vi "Autonomous Independent.vi"() -> ()   [LabVIEW 2013]
doc: "This VI is called when autonomous begins, and will automatically be terminated when autonomous ends. You can carry out timed or sensor driven robot movement independently without needing to return to the caller."
uses:
  Begin/Global Refnums.vi
  Begin/Global Variables.vi
  <vilib>/Rock Robotics/WPI/DriverStation/DriverStationLCD/WPI_DriverStationLCDLCDLine.ctl
panel:
  out "Index 2":i32
  # "Be sure to right-click and choose Data Operations>>Make Current Value default if you want to save the array values with the VI"
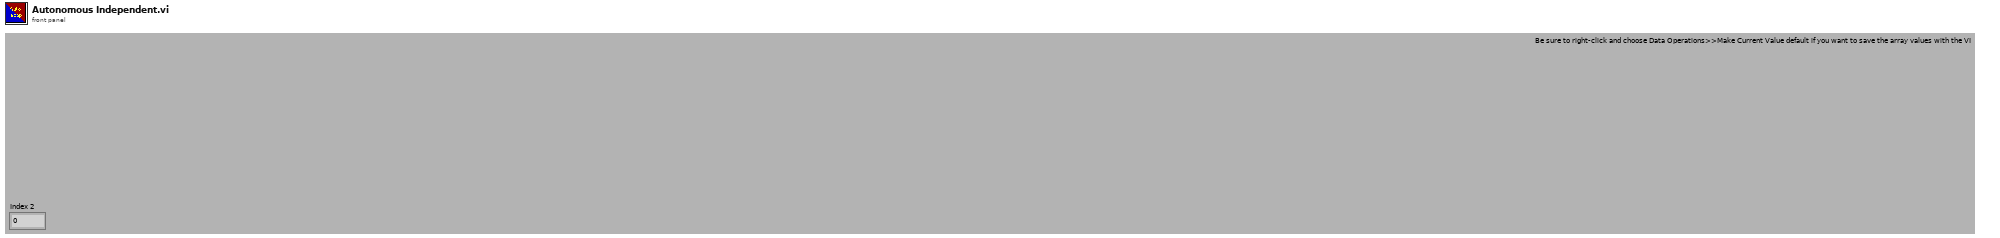
[diagram p1: front panel]
types:
  T1 = typedef "WPI_DriverStationLCDLCDLine.ctl" = enum16{"Main - Line 1", "User - Line 2", "User - Line 3", "User - Line 4", "User - Line 5", "User - Line 6"}
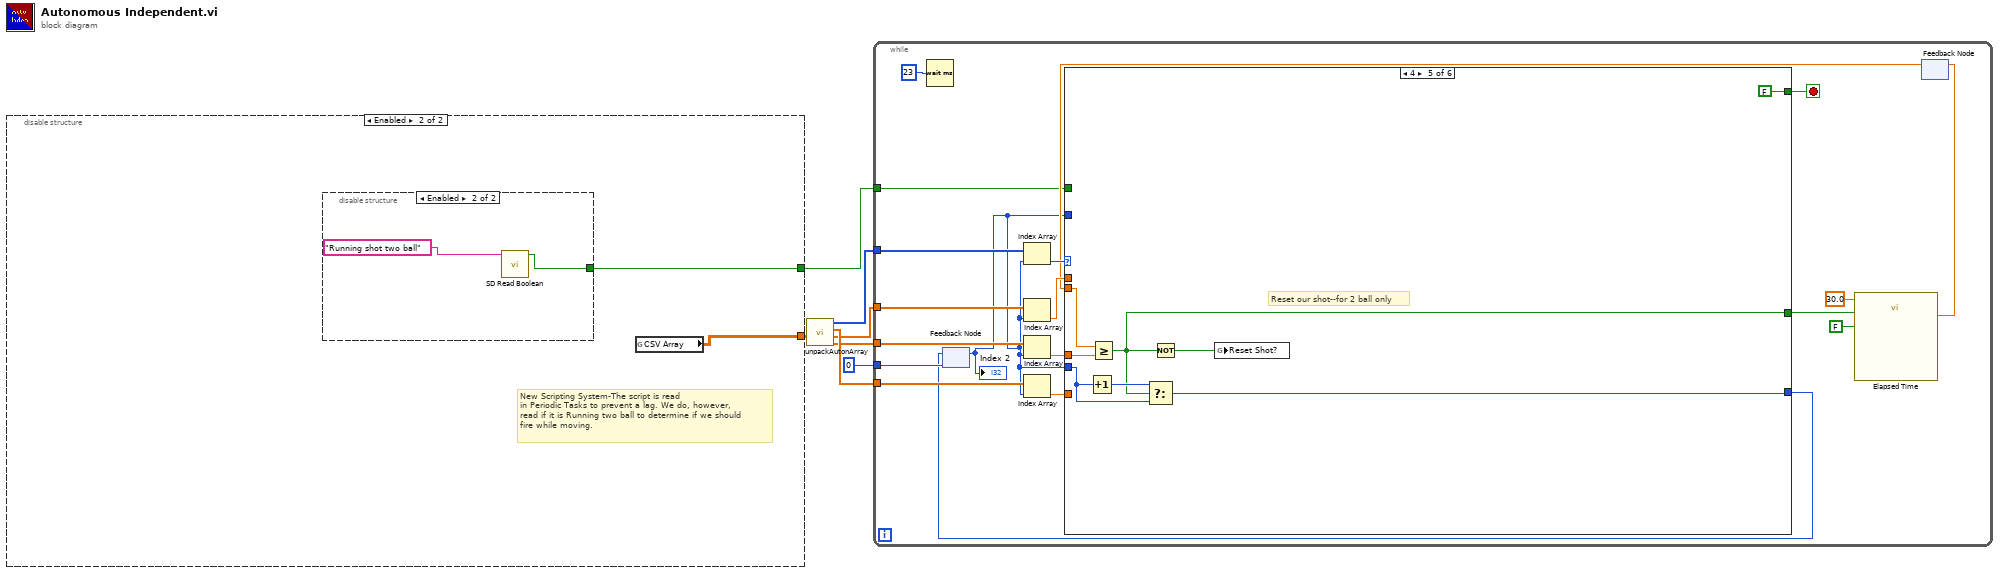
[diagram p0: block diagram]
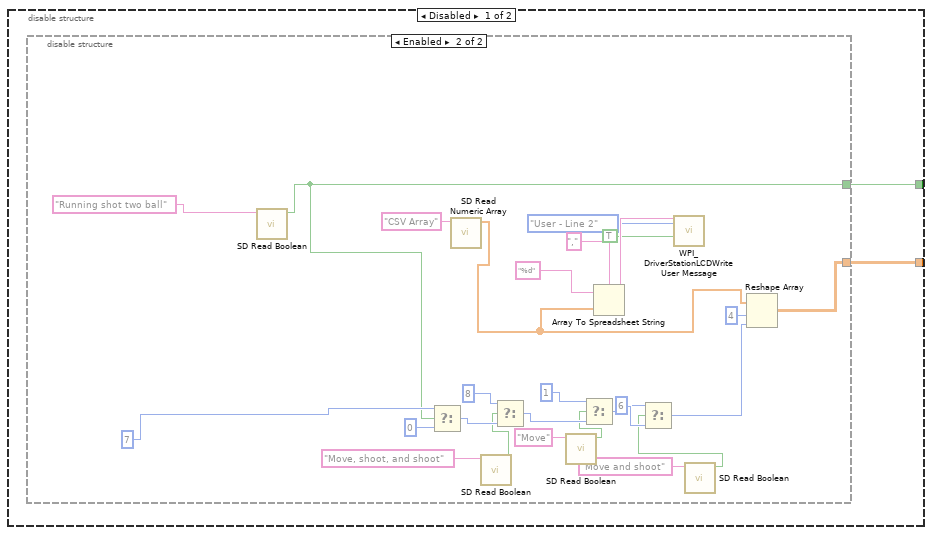
[diagram p2: hidden frame]
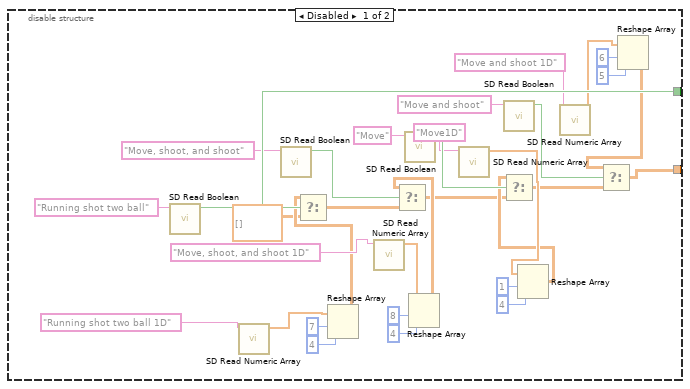
[diagram p3: hidden frame]
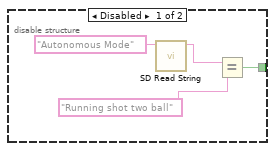
[diagram p4: hidden frame]
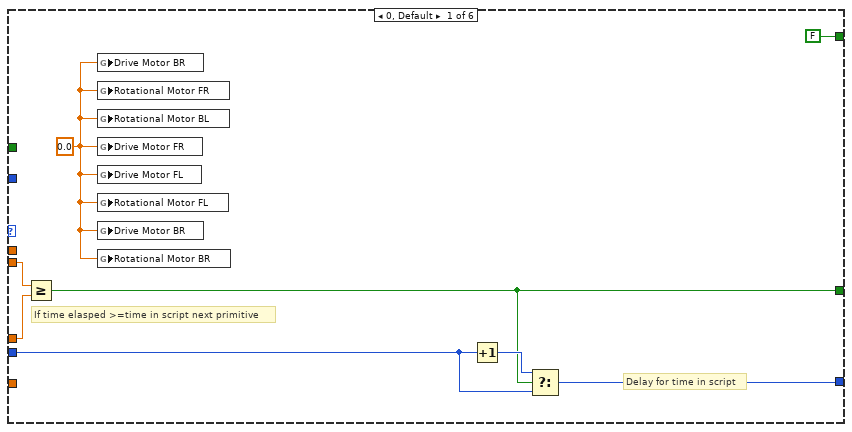
[diagram p5: hidden frame]
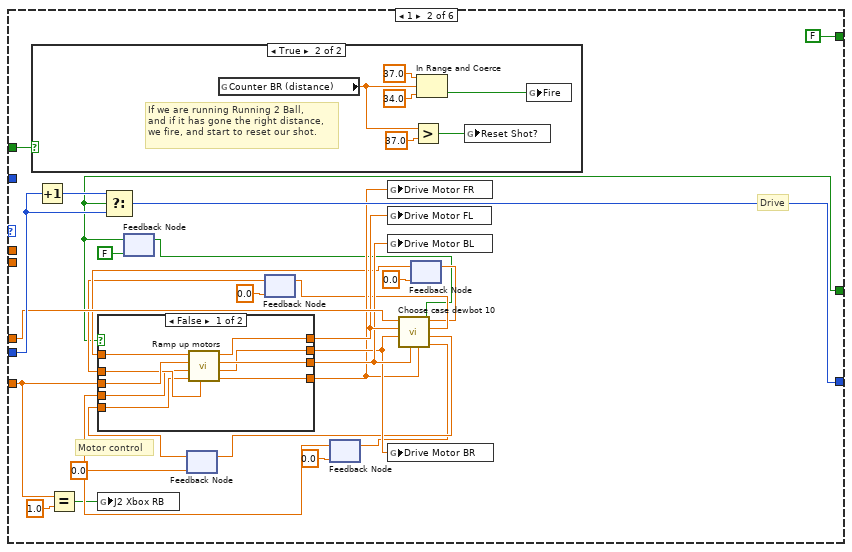
[diagram p6: hidden frame]
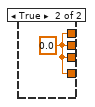
[diagram p8: hidden frame]
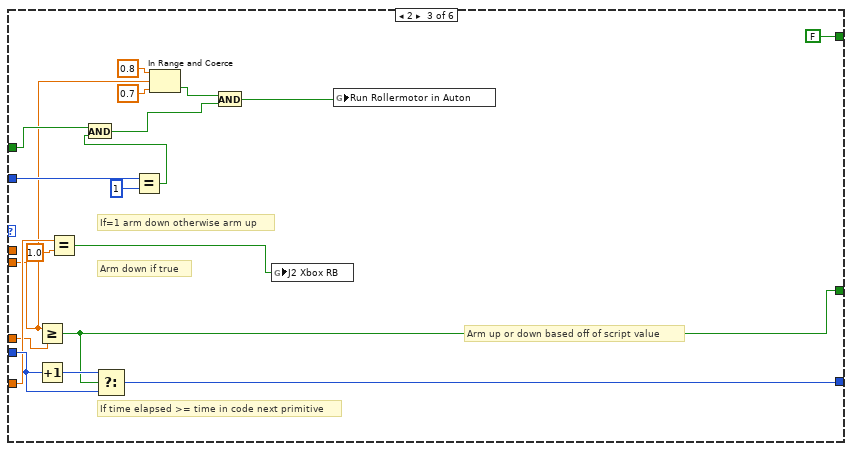
[diagram p9: hidden frame]
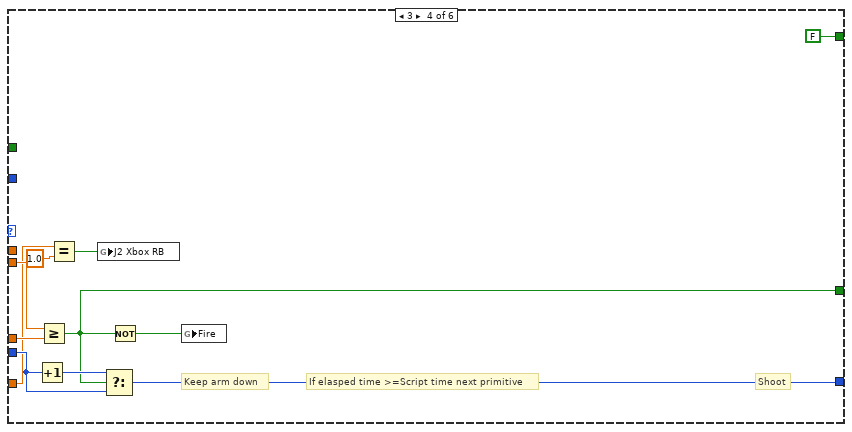
[diagram p10: hidden frame]
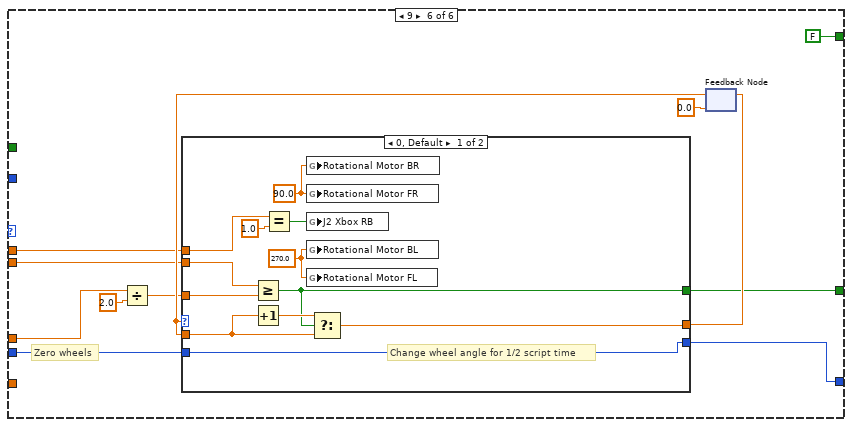
[diagram p11: hidden frame]
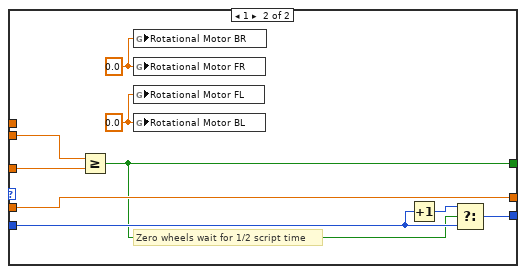
[diagram p12: hidden frame]
diagram:
  n1 = disable-structure shown="Enabled" {
    disable-tunnel: [w9 w69] -> w2
    disable-tunnel: [w8 w70] -> w1
    frame Disabled {
      n2 = disable-structure shown="Enabled" {
        disable-tunnel: [w42 w57] -> w9
        disable-tunnel: [w11 w49] -> w8
        frame Disabled {
          n3 = call <vilib>:"SD Read Boolean.vi"("Name"="Running shot two ball") -> ("Boolean"=w42:bool)  [unwired: 8 in, 2 out]
          n4 = call <vilib>:"SD Read Numeric Array.vi"("Name"="Running shot two ball 1D") -> ("Numeric Array"=w15:dbl[])  [unwired: 8 in, 2 out]
          n5 = call <vilib>:"SD Read Boolean.vi"("Name"="Move, shoot, and shoot") -> ("Boolean"=w35:bool)  [unwired: 8 in, 2 out]
          n6 = Reshape Array(w15, 7 ("dimension size"), 4 ("dimension size")) -> (w14:dbl[][])
          n7 = Select(t=w14, s=w42, f=dbl[][] []) -> (s? t:f=w13:dbl[][])
          n8 = call <vilib>:"SD Read Numeric Array.vi"("Name"="Move, shoot, and shoot 1D") -> ("Numeric Array"=w18:dbl[])  [unwired: 8 in, 2 out]
          n9 = call <vilib>:"SD Read Boolean.vi"("Name"="Move") -> ("Boolean"=w39:bool)  [unwired: 8 in, 2 out]
          n10 = Reshape Array(w18, 8 ("dimension size"), 4 ("dimension size")) -> (w17:dbl[][])
          n11 = Select(t=w17, s=w35, f=w13) -> (s? t:f=w16:dbl[][])
          n12 = call <vilib>:"SD Read Numeric Array.vi"("Name"="Move1D") -> ("Numeric Array"=w20:dbl[])  [unwired: 8 in, 2 out]
          n13 = call <vilib>:"SD Read Boolean.vi"("Name"="Move and shoot") -> ("Boolean"=w38:bool)  [unwired: 8 in, 2 out]
          n14 = Reshape Array(w20, 1 ("dimension size"), 4 ("dimension size")) -> (w19:dbl[][])
          n15 = Select(t=w19, s=w39, f=w16) -> (s? t:f=w12:dbl[][])
          n16 = call <vilib>:"SD Read Numeric Array.vi"("Name"="Move and shoot 1D") -> ("Numeric Array"=w30:dbl[])  [unwired: 8 in, 2 out]
          n17 = Reshape Array(w30, 6 ("dimension size"), 5 ("dimension size")) -> (w27:dbl[][])
          n18 = Select(t=w27, s=w38, f=w12) -> (s? t:f=w11:dbl[][])
        }
        frame Enabled {
          n19 = call <vilib>:"SD Read Boolean.vi"("Name"="Running shot two ball") -> ("Boolean"=w57:bool)  [unwired: 8 in, 2 out]
          n20 = Select(t=7 ("dimension size"), s=w57, f=0) -> (s? t:f=w63:i32)
          n21 = call <vilib>:"SD Read Numeric Array.vi"("Name"="CSV Array") -> ("Numeric Array"=w44:dbl[])  [unwired: 8 in, 2 out]
          n22 = call <vilib>:"SD Read Boolean.vi"("Name"="Move, shoot, and shoot") -> ("Boolean"=w52:bool)  [unwired: 8 in, 2 out]
          n23 = Select(t=8 ("dimension size"), s=w52, f=w63) -> (s? t:f=w61:i32)
          n24 = call <vilib>:"SD Read Boolean.vi"("Name"="Move") -> ("Boolean"=w54:bool)  [unwired: 8 in, 2 out]
          n25 = Select(t=1 ("dimension size"), s=w54, f=w61) -> (s? t:f=w60:i32)
          n26 = Array To Spreadsheet String(delimiter (Tab)=",", array=w44, 3:"%d" ("format string")) -> (spreadsheet string=w48:string)
          n27 = call <vilib>:"WPI_DriverStationLCDWrite User Message.vi"("line text"=w48, "line"=WPI_DriverStationLCDLCDLine."User - Line 2", "clear line before write (T)"=TRUE) -> ()  [unwired: 12 in, 1 out]
          n28 = call <vilib>:"SD Read Boolean.vi"("Name"="Move and shoot") -> ("Boolean"=w50:bool)  [unwired: 8 in, 2 out]
          n29 = Select(t=6, s=w50, f=w60) -> (s? t:f=w56:i32)
          n30 = Reshape Array(w44, 4 ("dimension size"), w56) -> (w49:dbl[][])
        }
      }
    }
    frame Enabled {
      # "New Scripting System-The script is read \nin Periodic Tasks to prevent a lag. We do, however,\nread if it is Running two ball to determine if we should \nfire while moving."
      n31 = disable-structure shown="Enabled" {
        disable-tunnel: [w71 w75] -> w69
        frame Disabled {
          n32 = call <vilib>:"SD Read String.vi"("Name"="Autonomous Mode") -> ("String"=w73:string)  [unwired: 8 in, 2 out]
          n33 = Equal?(x=w73, y="Running shot two ball") -> (x = y?=w71:bool)
        }
        frame Enabled {
          n34 = call <vilib>:"SD Read Boolean.vi"("Name"="Running shot two ball") -> ("Boolean"=w75:bool)  [unwired: 8 in, 2 out]
        }
      }
      n35 = global read "Global Refnums.vi" "CSV Array"() -> (w70:dbl[][])
    }
  }
  n36 = call "unpackAutonArray.vi"("all rows"=w1) -> ("Distance/time"=w3:dbl[], "Heading/Shoot angle"=w4:dbl[], "Power/Arm"=w5:dbl[], "Primitive"=w6:i16[])  [unwired: 6 in, 1 out]
  n37 = while {
    tunnel: w6 -> [w92]
    tunnel: w5 -> [w91]
    tunnel: w4 -> [w90]
    tunnel: w3 -> [w89]
    tunnel: 0 -> [w88]
    tunnel: w2 -> [w78]
    stop <- w93 stop-if-true
    n38 = Wait (ms)(milliseconds to wait=u32 23) -> ()  [unwired: 1 out]
    n39 = feedback #1(w88) -> (w77:i32)
    "Index 2" <- w77
    n40 = Index Array(array=w92, index=w77) -> (element=w95:i16)
    n41 = Index Array(array=w90, index=w77) -> (element=w84:dbl)
    n42 = Index Array(array=w89, index=w77) -> (element=w86:dbl)
    n43 = Index Array(array=w91, index=w77) -> (element=w85:dbl)
    n44 = feedback #2() -> (w81:dbl)  [unwired: 1 in]
    n45 = case shown="4" w95 {
      tunnel: w84 -> [_ _ _ _ _ w192]
      tunnel: w85 -> [_ w106 w160 w169 _ _]
      tunnel: [w102 w130 w163 w175 w183 w194] -> w87
      tunnel: w86 -> [w99 w128 w156 w173 w181 w190]
      tunnel: [FALSE ("Next primitive?") FALSE ("Next primitive?") FALSE ("Next primitive?") FALSE ("Next primitive?") FALSE ("Next primitive?") FALSE ("Next primitive?")] -> w93
      tunnel: w77 -> [w101 w129 w164 w177 w184 w195]
      tunnel: [w98 w110 w161 w171 w178 w191] -> w83
      tunnel: w81 -> [w100 _ w149 w172 w180 w187]
      tunnel: w78 -> [_ w104 w159 _ _ _]
      tunnel: w77 -> [_ _ w152 _ _ _]
      frame 0, Default {
        w97 = 0.0
        # "Delay for time in script"
        # "If time elasped >=time in script next primitive"
        n46 = Greater Or Equal?(x=w100, y=w99) -> (x >= y?=w98:bool)
        n47 = global write "Global Variables.vi" "Drive Motor BR"(w97) -> ()
        n48 = global write "Global Variables.vi" "Rotational Motor FR"(w97) -> ()
        n49 = global write "Global Variables.vi" "Rotational Motor BL"(w97) -> ()
        n50 = global write "Global Variables.vi" "Drive Motor FR"(w97) -> ()
        n51 = global write "Global Variables.vi" "Drive Motor FL"(w97) -> ()
        n52 = global write "Global Variables.vi" "Rotational Motor FL"(w97) -> ()
        n53 = global write "Global Variables.vi" "Drive Motor BR"(w97) -> ()
        n54 = global write "Global Variables.vi" "Rotational Motor BR"(w97) -> ()
        n55 = Increment(x=w101) -> (x+1=w103:i32)
        n56 = Select(t=w103, s=w98, f=w101) -> (s? t:f=w102:i32)
      }
      frame 1 {
        # "Motor control"
        # "Drive"
        n57 = case shown="True" w104 {
          frame False {
          }
          frame True {
            # "If we are running Running 2 Ball,\nand if it has gone the right distance,\nwe fire, and start to reset our shot."
            n58 = global read "Global Refnums.vi" "Counter BR (distance)"() -> (w134:dbl)
            n59 = Greater?(x=w134, y=37.0) -> (0:w132:bool)
            n60 = In Range and Coerce(upper limit=37.0, x=w134, lower limit=34.0) -> (In Range?=w135:bool)  [unwired: 1 out]
            n61 = global write "Global Refnums.vi" "Reset Shot?"(w132) -> ()
            n62 = global write "Global Refnums.vi" "Fire"(w135) -> ()
          }
        }
        n63 = Increment(x=w129) -> (x+1=w131:i32)
        n64 = Equal?(x=w106, y=1.0) -> (x = y?=w107:bool)
        n65 = global write "Global Variables.vi" "J2 Xbox RB"(w107) -> ()
        n66 = feedback #3(FALSE ("Next primitive?")) -> (w110:bool)
        n67 = Select(t=w131, s=w110, f=w129) -> (s? t:f=w130:i32)
        n68 = feedback #4(0.0 ("Last BL motor value")) -> (w119:dbl)
        n69 = feedback #5(0.0 ("Last BR motor value")) -> (w121:dbl)
        n70 = feedback #6(0.0 ("Last FR motor value")) -> (w117:dbl)
        n71 = feedback #7(0.0 ("Last FL motor value")) -> (w123:dbl)
        n72 = case shown="False" w110 {
          tunnel: w106 -> [w146 _]
          tunnel: [w145 w147] -> w127
          tunnel: [w144 w147] -> w126
          tunnel: [w143 w147] -> w125
          tunnel: [w142 w147] -> w124
          tunnel: w123 -> [w141 _]
          tunnel: w121 -> [w140 _]
          tunnel: w119 -> [w139 _]
          tunnel: w117 -> [w138 _]
          frame False {
            n73 = call "Ramp up motors.vi"("Last BR motor value"=w140, "Last BL motor value"=w139, "Last FR motor value"=w138, "Set motor value"=w146, "Last FL motor value"=w141) -> ("Next FR motor value"=w142:dbl, "Next BR motor value"=w143:dbl, "Next BL motor value"=w144:dbl, "Next FL motor value"=w145:dbl)  [unwired: 3 in]
          }
          frame True {
            w147 = 0.0 ("Next FL motor value")
          }
        }
        n74 = global write "Global Variables.vi" "Drive Motor FR"(w124) -> ()
        n75 = global write "Global Variables.vi" "Drive Motor FL"(w127) -> ()
        n76 = global write "Global Variables.vi" "Drive Motor BL"(w126) -> ()
        n77 = global write "Global Variables.vi" "Drive Motor BR"(w125) -> ()
        n78 = call "Choose case dewbot 10.vi"("Next FR motor value"=w124, "Next BL motor value"=w126, "Next BR motor value"=w125, "Next FL motor value"=w127, "Set Tac value"=w128) -> ("Last FR motor value"=w118:dbl, "Last BL motor value"=w120:dbl, "Last BR motor value"=w122:dbl, "Last FL motor value"=w112:dbl, "Next primitive?"=w111:bool)  [unwired: 2 in]
        n79 = feedback-in #3(w111) -> ()
        n80 = feedback-in #4(w120) -> ()
        n81 = feedback-in #5(w122) -> ()
        n82 = feedback-in #6(w118) -> ()
        n83 = feedback-in #7(w112) -> ()
      }
      frame 2 {
        # "Arm down if true"
        # "If time elapsed >= time in code next primitive"
        # "If=1 arm down otherwise arm up"
        # "Arm up or down based off of script value"
        n84 = Greater Or Equal?(x=w149, y=w156) -> (x >= y?=w161:bool)
        n85 = Increment(x=w164) -> (x+1=w165:i32)
        n86 = Equal?(x=w160, y=1.0) -> (x = y?=w153:bool)
        n87 = Select(t=w165, s=w161, f=w164) -> (s? t:f=w163:i32)
        n88 = Equal?(x=w152, y=1) -> (x = y?=w148:bool)
        n89 = And(x=w159, y=w148) -> (x .and. y?=w154:bool)
        n90 = In Range and Coerce(upper limit=0.8, x=w149, lower limit=0.7) -> (In Range?=w155:bool)  [unwired: 1 out]
        n91 = And(x=w155, y=w154) -> (x .and. y?=w150:bool)
        n92 = global write "Global Variables.vi" "J2 Xbox RB"(w153) -> ()
        n93 = global write "Global Refnums.vi" "Run Rollermotor in Auton"(w150) -> ()
      }
      frame 3 {
        # "Keep arm down"
        # "If elasped time >=Script time next primitive"
        # "Shoot"
        n94 = Increment(x=w177) -> (x+1=w176:i32)
        n95 = Greater Or Equal?(x=w172, y=w173) -> (x >= y?=w171:bool)
        n96 = Equal?(x=w169, y=1.0) -> (x = y?=w167:bool)
        n97 = global write "Global Variables.vi" "J2 Xbox RB"(w167) -> ()
        n98 = Select(t=w176, s=w171, f=w177) -> (s? t:f=w175:i32)
        n99 = Not(x=w171) -> (.not. x?=w174:bool)
        n100 = global write "Global Refnums.vi" "Fire"(w174) -> ()
      }
      frame 4 {
        # "Reset our shot--for 2 ball only"
        n101 = Increment(x=w184) -> (x+1=w185:i32)
        n102 = Greater Or Equal?(x=w180, y=w181) -> (x >= y?=w178:bool)
        n103 = Select(t=w185, s=w178, f=w184) -> (s? t:f=w183:i32)
        n104 = Not(x=w178) -> (.not. x?=w179:bool)
        n105 = global write "Global Refnums.vi" "Reset Shot?"(w179) -> ()
      }
      frame 9 {
        # "Zero wheels"
        n106 = Divide(x=w190, y=2.0) -> (x/y=w189:dbl)
        n107 = feedback #8(0.0) -> (w196:dbl)
        n108 = case shown="0, Default" w196 {
          tunnel: [w201 w213] -> w197
          tunnel: w196 -> [w202 w213]
          tunnel: w195 -> [w204 w214]
          tunnel: [w204 w215] -> w194
          tunnel: w192 -> [w205 _]
          tunnel: w189 -> [w199 w211]
          tunnel: [w200 w212] -> w191
          tunnel: w187 -> [w198 w210]
          frame 0, Default {
            w207 = 270.0 ("Rotational Motor FL")
            w206 = 90.0 ("Rotational Motor FR")
            # "Change wheel angle for 1/2 script time"
            n109 = Greater Or Equal?(x=w198, y=w199) -> (x >= y?=w200:bool)
            n110 = Increment(x=w202) -> (x+1=w203:dbl)
            n111 = Equal?(x=w205, y=1.0) -> (x = y?=w209:bool)
            n112 = global write "Global Variables.vi" "Rotational Motor BR"(w206) -> ()
            n113 = global write "Global Variables.vi" "Rotational Motor FR"(w206) -> ()
            n114 = global write "Global Variables.vi" "J2 Xbox RB"(w209) -> ()
            n115 = global write "Global Variables.vi" "Rotational Motor BL"(w207) -> ()
            n116 = global write "Global Variables.vi" "Rotational Motor FL"(w207) -> ()
            n117 = Select(t=w203, s=w200, f=w202) -> (s? t:f=w201:dbl)
          }
          frame 1 {
            w218 = 0.0 ("Rotational Motor BL")
            w217 = 0.0
            # "Zero wheels wait for 1/2 script time"
            n118 = Greater Or Equal?(x=w210, y=w211) -> (x >= y?=w212:bool)
            n119 = global write "Global Variables.vi" "Rotational Motor BR"(w217) -> ()
            n120 = global write "Global Variables.vi" "Rotational Motor FR"(w217) -> ()
            n121 = global write "Global Variables.vi" "Rotational Motor FL"(w218) -> ()
            n122 = global write "Global Variables.vi" "Rotational Motor BL"(w218) -> ()
            n123 = Increment(x=w214) -> (x+1=w216:i32)
            n124 = Select(t=w216, s=w212, f=w214) -> (s? t:f=w215:i32)
          }
        }
        n125 = feedback-in #8(w197) -> ()
      }
    }
    n126 = feedback-in #1(w87) -> ()
    n127 = call "Elapsed Time"("Time Target (s)"=30.0, "Reset"=w83, "Auto Reset"=FALSE) -> ("Elapsed Time (s)"=w79:dbl)  [unwired: 9 in, 7 out]
    n128 = feedback-in #2(w79) -> ()
  }
